vi "Unmarshal.vi"(8 "error in (no error)":errorcluster, 10 "Buffer":u8[](array[numeric]), 11 "int32 in":refnum<class "int64.lvclass">) -> (0 "error out":errorcluster, 2 "Buffer Count":i32=8, 3 "int32 out":refnum<class "int64.lvclass">)   [LabVIEW 2020, in "Protobuf RAW.lvlib" / "int64.lvclass"]
uses:
  int64.lvclass
  int64.lvclass/int64.ctl
  Protobuf RAW.lvlib
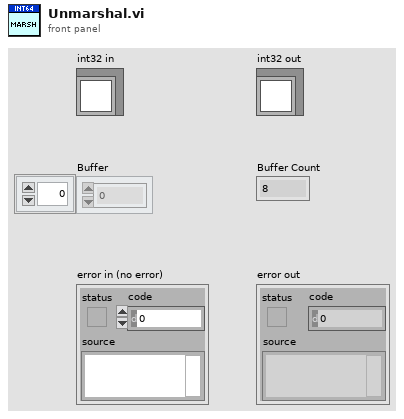
[diagram p1: front panel]
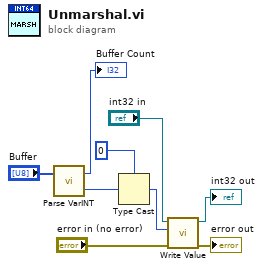
[diagram p0: block diagram]
diagram:
  n1 = call "Parse VarINT.vi"("Buffer"="Buffer") -> ("Numeric"=w6:u64, "Bytes"=→"Buffer Count":i32)  [unwired: 1 in]
  n2 = Type Cast(type=i64 0 ("Numeric"), x=w6) -> (*(type *) &x=w1:i64)
  n3 = call "Write Value.vi"("error in (no error)"="error in (no error)", "Value"=w1, "int32 in"="int32 in") -> ("error out"=→"error out":errorcluster, "int32 out"=→"int32 out":refnum<class "int64.lvclass">)  [unwired: 7 in]
